vi "主vi.vi"() -> ()   [LabVIEW 2015]
panel:
  in  "下拉列表":u16(ring)
  in  "选项卡3":enum32{"选项卡 1", "选项卡 2"}(tab)
  in  "选项卡2":enum32{"选项卡 1", "选项卡 2"}(tab)
  in  "选项卡1":enum32{"111", "222"}(tab) caption="选项卡控件"
  in  "字符串":string
  in  "布尔":bool
  in  "数值":dbl
  out "用户名的顺序":u16
  out "用户类别":u8
  out "管理人员1+密码":string[][](array[string])
  out "操作人员0+密码":string[][](array[string])
  out "密码文件路径":path
  in  "管理":bool
  in  "取消":bool
  out "当前用户类别":string
  out "当前用户名":string
  # "管理人员可以玩\n操作人员不让玩"
  # "界面乱，临时调试，\n最后有些要隐藏的"
  # "11111111111"
  # "管理员可以看到22222222"
  # "管理员可以看到"
  # "22222222"
  # "11111111"
  # "22222222"
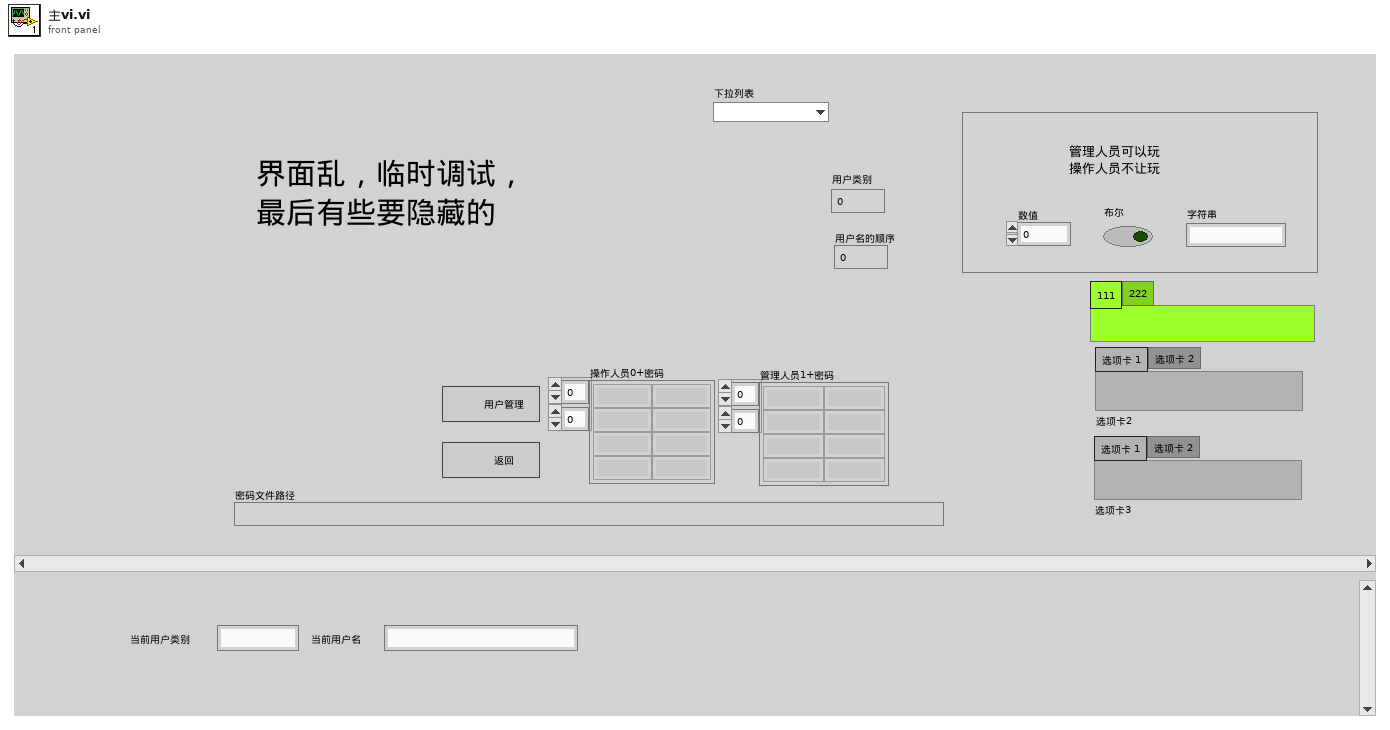
[diagram p1: front panel]
types:
  T1 = enum8{"Enabled", "Disabled", "Disabled and Grayed Out"}
  T2 = enum32{"invalid app kind", "Development System", "Run Time System", "Student Edition", "Embedded LabVIEW", "Evaluation", "Custom"}
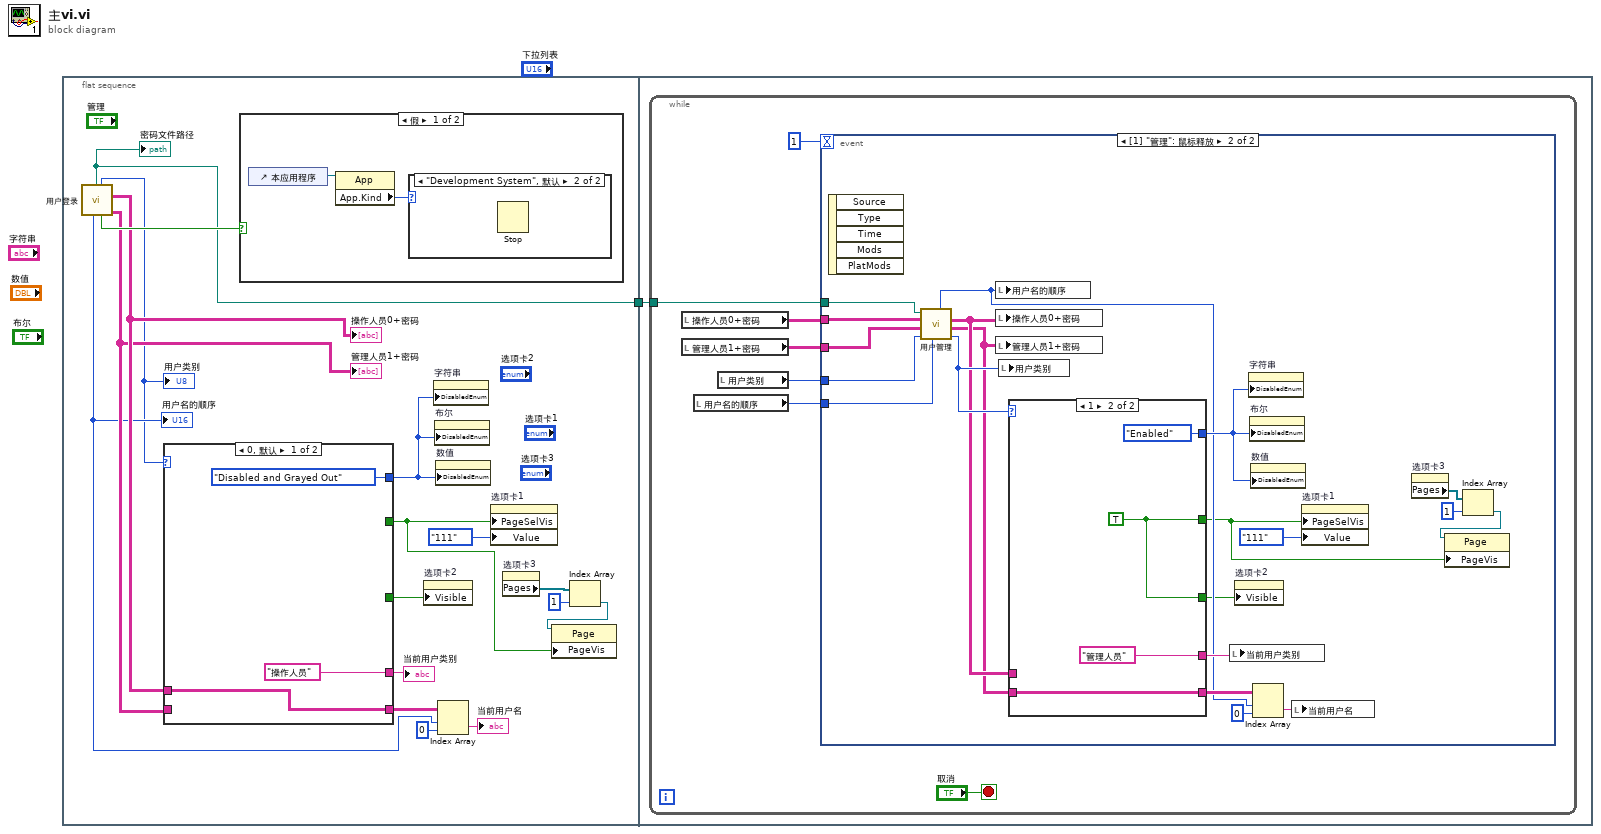
[diagram p0: block diagram]
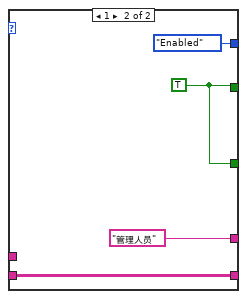
[diagram p2: hidden frame]
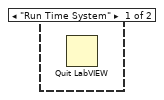
[diagram p3: hidden frame]
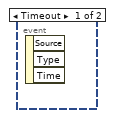
[diagram p5: hidden frame]
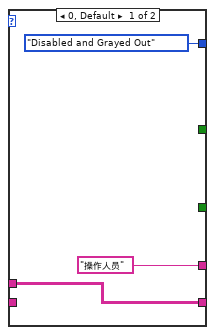
[diagram p6: hidden frame]
diagram:
  n1 = flat-sequence {
    tunnel: [w13] -> w1
    tunnel: w1 -> [w28]
    frame #0 {
      n2 = call "用户登录.vi"() -> ("管理人员1+密码"=w11:string[][], "操作人员0+密码"=w12:string[][], "T正常-F错误"=w18:bool, "用户类别_out"=w9:u8, "用户名的顺序out"=w10:u16, "密码文件路径"=w13:path)  [unwired: 4 in, 2 out]
      "密码文件路径" <- w13
      "操作人员0+密码" <- w12
      "管理人员1+密码" <- w11
      "用户名的顺序" <- w10
      "用户类别" <- w9
      n3 = case shown="0, 默认" w9 {
        tunnel: ["操作人员" "管理人员"] -> w17
        tunnel: w11 -> [_ w24]
        tunnel: [w20 w24] -> w16
        tunnel: w12 -> [w20 _]
        tunnel: [T1."Disabled and Grayed Out" ("禁用") T1."Enabled" ("禁用")] -> w8
        tunnel: [_ w22] -> w2
        tunnel: [_ w22] -> w6
        frame 0, Default {
        }
        frame 1 {
          w22 = TRUE
        }
      }
      "当前用户类别" <- w17
      n4 = case shown="假" w18 {
        frame False {
          n5 = control-ref of="本应用程序"() -> (w26:refnum<vi>)
          n6 = property class="App"(reference=w26) -> ("App.Kind"=w27:T2)  [unwired: 1 in, 2 out]
          n7 = case shown="\"Development System\", 默认" w27 {
            frame "Run Time System" {
              n8 = Quit LabVIEW() -> ()  [unwired: 1 in]
            }
            frame "Development System", Default {
              n9 = Stop() -> ()  [unwired: 1 in]
            }
          }
        }
        frame True {
        }
      }
      n10 = property on="选项卡2" class="TabCtl (严格)"("Visible"=w6) -> ()  [unwired: 2 in, 2 out]
      n11 = property on="字符串" class="Str"("DisabledEnum"=w8) -> ()  [unwired: 2 in, 2 out]
      n12 = property on="布尔" class="Bool (严格)"("DisabledEnum"=w8) -> ()  [unwired: 2 in, 2 out]
      n13 = property on="数值" class="DigNum (严格)"("DisabledEnum"=w8) -> ()  [unwired: 2 in, 2 out]
      n14 = Index Array(array=w16, index (row)=w10, index (col)=0 ("禁用的索引 (列)")) -> (element=→"当前用户名":string)
      n15 = property on="选项卡1" class="TabCtl (严格)"("PageSelVis"=w2, "Value"=enum32{"111", "222"}."111" ("选项卡控件")) -> ()  [unwired: 2 in, 2 out]
      n16 = property on="选项卡3" class="TabCtl (严格)"() -> ("Pages"=w5:refnum<vi>[])  [unwired: 2 in, 2 out]
      n17 = Index Array(array=w5, index=1 ("索引")) -> (element=w3:refnum<vi>)
      n18 = property class="Page"(reference=w3, "PageVis"=w2) -> ()  [unwired: 1 in, 2 out]
    }
    frame #1 {
      n19 = while {
        tunnel: w28 -> [w33]
        stop <- "取消" stop-if-true
        n20 = local read "操作人员0+密码"() -> (w31:string[][])
        n21 = local read "管理人员1+密码"() -> (w30:string[][])
        n22 = local read "用户名的顺序"() -> (w29:u16)
        n23 = local read "用户类别"() -> (w32:u8)
        n24 = event shown="[1] \"管理\": 鼠标释放" {
          selector: _ -> [_ _]
          dyn-events: _ -> [_ _]
          timeout: 1 -> [_ _]
          tunnel: w33 -> [_ w55]
          tunnel: w31 -> [_ w54]
          tunnel: w32 -> [_ w53]
          tunnel: w30 -> [_ w52]
          tunnel: w29 -> [_ w51]
          event Timeout {
            n25 = event-data() -> ()  [unwired: 1 in, 3 out]
          }
          event "管理": Mouse Up {
            n26 = event-data() -> ()  [unwired: 1 in, 5 out]
            n27 = call "用户管理.vi"("用户名的顺序"=w51, "用户类别"=w53, "管理人员1+密码"=w52, "操作人员0+密码"=w54, "密码文件路径"=w55) -> ("用户类别-out"=w47:u8, "管理人员1+密码-out"=w43:string[][], "操作人员0+密码-out"=w44:string[][], "用户名的顺序-out"=w42:u16)  [unwired: 2 in, 1 out]
            n28 = local write "用户名的顺序"(w42) -> ()
            n29 = local write "操作人员0+密码"(w44) -> ()
            n30 = local write "管理人员1+密码"(w43) -> ()
            n31 = local write "用户类别"(w47) -> ()
            n32 = case shown="1" w47 {
              tunnel: ["操作人员" "管理人员"] -> w46
              tunnel: w43 -> [_ w61]
              tunnel: [w57 w61] -> w48
              tunnel: w44 -> [w57 _]
              tunnel: [T1."Disabled and Grayed Out" ("禁用") T1."Enabled" ("禁用")] -> w50
              tunnel: [_ w59] -> w37
              tunnel: [_ w59] -> w40
              frame 0, Default {
              }
              frame 1 {
                w59 = TRUE
              }
            }
            n33 = local write "当前用户类别"(w46) -> ()
            n34 = property on="选项卡2" class="TabCtl (严格)"("Visible"=w40) -> ()  [unwired: 2 in, 2 out]
            n35 = property on="字符串" class="Str"("DisabledEnum"=w50) -> ()  [unwired: 2 in, 2 out]
            n36 = property on="布尔" class="Bool (严格)"("DisabledEnum"=w50) -> ()  [unwired: 2 in, 2 out]
            n37 = property on="数值" class="DigNum (严格)"("DisabledEnum"=w50) -> ()  [unwired: 2 in, 2 out]
            n38 = Index Array(array=w48, index (row)=w42, index (col)=0 ("禁用的索引 (列)")) -> (element=w45:string)
            n39 = local write "当前用户名"(w45) -> ()
            n40 = property on="选项卡1" class="TabCtl (严格)"("PageSelVis"=w37, "Value"=enum32{"111", "222"}."111" ("选项卡控件")) -> ()  [unwired: 2 in, 2 out]
            n41 = property on="选项卡3" class="TabCtl (严格)"() -> ("Pages"=w38:refnum<vi>[])  [unwired: 2 in, 2 out]
            n42 = Index Array(array=w38, index=1 ("索引")) -> (element=w36:refnum<vi>)
            n43 = property class="Page"(reference=w36, "PageVis"=w37) -> ()  [unwired: 1 in, 2 out]
          }
        }
      }
    }
  }
